vi "New Device Dialog.vi"(8 "error in (no error)":errorcluster, 11 "Configuration in":refnum<class "Configuration.lvclass">) -> (0 "error out":errorcluster, 1 "Class Path":path, 2 "Cancelled?":bool, 3 "Configuration out":refnum<class "Configuration.lvclass">)   [LabVIEW 2023, in "Configuration.lvlib" / "Configuration.lvclass"]
uses:
  Library/Configuration.lvclass
  Library/Configuration.lvclass/Configuration.ctl
panel:
  in  "Cancel":bool
  in  "Ok":bool
  in  "Model":u16(ring) items=["--- Select Device Model ---"]
  in  "Category":u16(ring) items=["--- Select Device Category ---", "ANALOGINPUT", "POWERSUPPLY"]
  in  "Device":string
  # "Enter a name for the device, select a category, and then select a model"
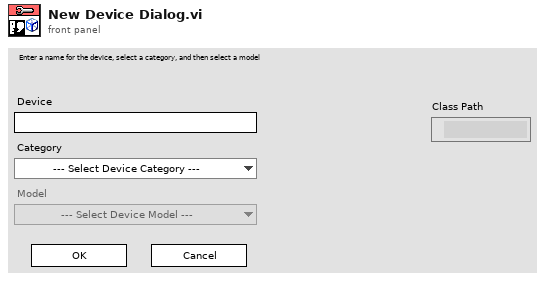
[diagram p1: front panel]
types:
  T1 = enum8{"Enabled", "Disabled", "Disabled and Grayed Out"}
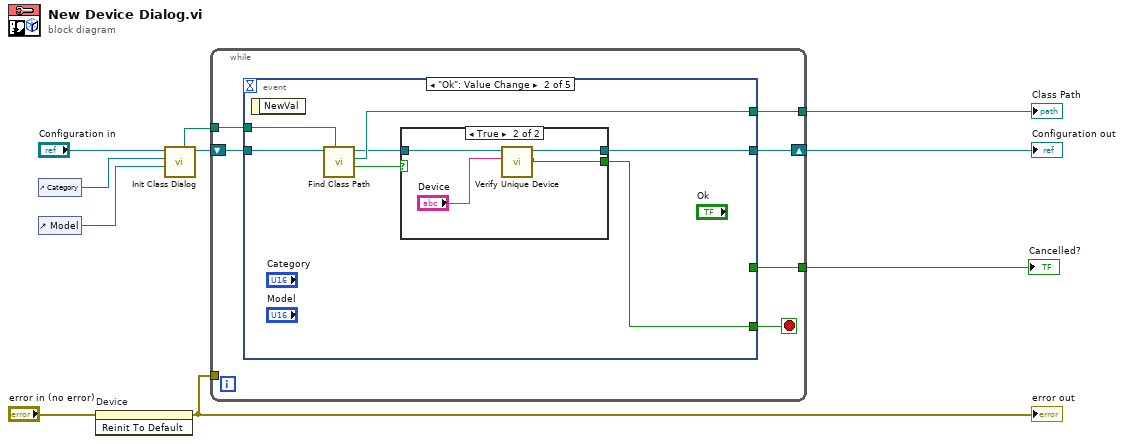
[diagram p0: block diagram]
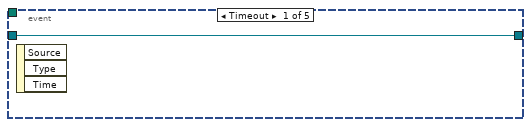
[diagram p2: hidden frame]
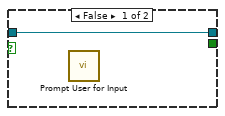
[diagram p3: hidden frame]
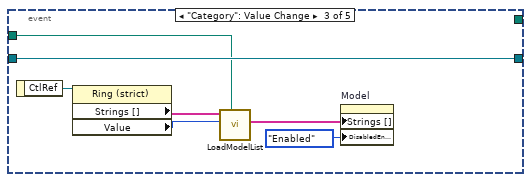
[diagram p4: hidden frame]
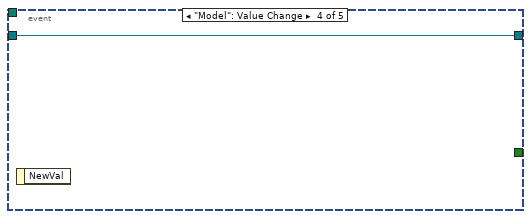
[diagram p5: hidden frame]
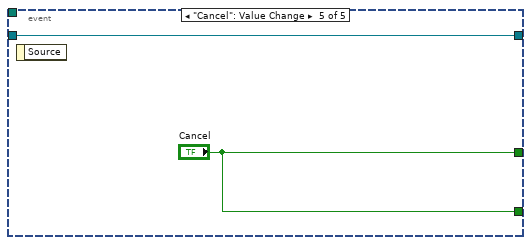
[diagram p6: hidden frame]
diagram:
  n1 = control-ref of="Category"() -> (w5:refnum<vi>)
  n2 = control-ref of="Model"() -> (w4:refnum<vi>)
  n3 = invoke on="Device" class="Str" method="Reinit To Default"(error in="error in (no error)") -> (error out=w1:errorcluster)  [unwired: 2 in, 2 out]
  "error out" <- w1
  n4 = call "Init Class Dialog.vi"("ModelRef"=w4, "CategoryRef"=w5, "Configuration in"="Configuration in") -> ("Configuration out"=w7:refnum<class "Configuration.lvclass">, "Base Path"=w6:path)  [unwired: 6 in, 1 out]
  n5 = while {
    shift-right: [w15] -> w10
    shift-left: w7 -> [w16]
    tunnel: [w13] -> w9
    tunnel: w6 -> [w12]
    tunnel: [w11] -> w3
    tunnel: w1 -> [_]
    stop <- w14 stop-if-true
    n6 = event shown="[1] \"Ok\": Value Change" {
      selector: _ -> [_ _ _ _ _]
      dyn-events: _ -> [_ _ _ _ _]
      timeout: _ -> [_ _ _ _ _]
      tunnel: w16 -> [w17 w22 w36 w37 w39]
      tunnel: [w17 w19 w36 w37 w39] -> w15
      tunnel: [_ w18 _ _ "Cancel"] -> w14
      tunnel: [_ _ _ _ "Cancel"] -> w13
      tunnel: w12 -> [_ w24 w31 _ _]
      tunnel: [_ w23 _ _ _] -> w11
      event Timeout {
        n7 = event-data() -> ()  [unwired: 1 in, 3 out]
      }
      event "Ok": Value Change {
        n8 = event-data() -> ()  [unwired: 1 in, 1 out]
        n9 = call "Find Class Path.vi"("basepath"=w24, "Configuration in"=w22) -> ("LegalClass"=w21:bool, "Class Path"=w23:path, "Configuration out"=w20:refnum<class "Configuration.lvclass">)  [unwired: 6 in, 1 out]
        n10 = case shown="True" w21 {
          tunnel: w20 -> [w25 w28]
          tunnel: [w25 w27] -> w19
          tunnel: [_ w26] -> w18
          frame False {
            n11 = call "Prompt User for Input"() -> ()  [unwired: 18 in, 2 out]
          }
          frame True {
            n12 = call "Verify Unique Device.vi"("Device"="Device", "Configuration in"=w28) -> ("Name Added"=w26:bool, "Configuration out"=w27:refnum<class "Configuration.lvclass">)  [unwired: 7 in, 1 out]
          }
        }
      }
      event "Category": Value Change {
        n13 = event-data() -> ("CtlRef"=w34:refnum<vi>)  [unwired: 1 in]
        n14 = property class="Ring (strict)"(reference=w34) -> ("Strings []"=w33:string[], "Value"=w32:u16)  [unwired: 1 in, 2 out]
        n15 = call "LoadModelList.vi"("base path"=w31, "Value"=w32, "Strings []"=w33) -> ("Model Strings"=w30:string[])  [unwired: 8 in]
        n16 = property on="Model" class="Ring (strict)"("Strings []"=w30, "DisabledEnum"=T1."Enabled" ("Disabled")) -> ()  [unwired: 2 in, 2 out]
      }
      event "Model": Value Change {
        n17 = event-data() -> ()  [unwired: 1 in, 1 out]
      }
      event "Cancel": Value Change {
        n18 = event-data() -> ()  [unwired: 1 in, 1 out]
      }
    }
  }
  "Configuration out" <- w10
  "Cancelled?" <- w9
  "Class Path" <- w3
